vi "G#Interface_ClassToSpecificInterface.vi"(2 "reference in":refnum<class "G#Object.lvclass">, 4 "error in (no error)":errorcluster, 12 "target interface":refnum<class "G#Interface.lvclass">, 14 "autolocate?(F)":bool) -> (22 "interface reference out":refnum<class "G#Interface.lvclass">, 24 "error out":errorcluster)   [LabVIEW 2020, in "G#Interface.lvclass"]
doc: "Casts an ordinary G#Object reference to the specified G#Interface reference."
uses:
  G#Interface.lvclass
  G#Object/G#Object.lvclass
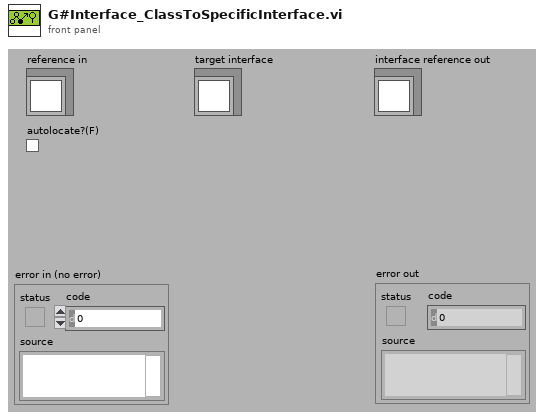
[diagram p1: front panel]
types:
  T1 = typedef "G#Object.lvclass/G#Object_ClassHierarchy.ctl" = cluster{"ClassName":string, "FullClassName":string, "ClassPath":path, "IsLeaf":bool}
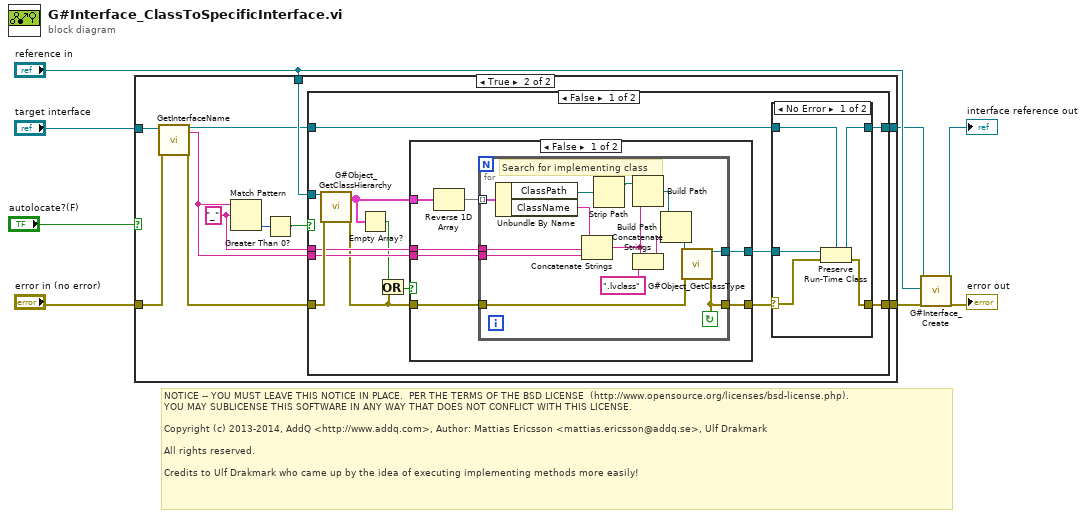
[diagram p0: block diagram]
diagram:
  # "NOTICE -- YOU MUST LEAVE THIS NOTICE IN PLACE.  PER THE TERMS OF THE BSD LICENSE  (http://www.opensource.org/licenses/bsd-license.php).\nYOU MAY SUBLICENSE THIS SOFTWARE IN ANY WAY THAT DOES NOT CONFLICT WITH THIS LICENSE.\n\nCopyright (c) 2013-2014, AddQ <http://www.addq.com>, Author: Mattias Ericsson <mattias.ericsson@addq.se>, Ulf Drakmark\n\nAll rights reserved.\n\nCredits to Ulf Drakmark who came up by the idea of executing implementing methods more easily!"
  n1 = case shown="True" "autolocate?(F)" {
    tunnel: "target interface" -> [w10 w21]
    tunnel: "error in (no error)" -> [w9 w20]
    tunnel: "reference in" -> [_ w19]
    tunnel: [w9 w18] -> w3
    tunnel: [w10 w17] -> w2
    frame False {
    }
    frame True {
      w13 = "_" ("regular expression")
      n2 = call-dynamic "GetInterfaceName.vi"("reference in"=w21, "error in (no error)"=w20) -> ("reference out"=w11:refnum<class "G#Interface.lvclass">, "interface name"=w12:string, "error out"=w15:errorcluster)  [unwired: 13 in, 2 out]
      n3 = Match Pattern(string=w12, regular expression=w13) -> (offset past match=w16:i32)  [unwired: 1 in, 3 out]
      n4 = Greater Than 0?(x=w16) -> (x > 0?=w14:bool)
      n5 = case shown="False" w14 {
        tunnel: w19 -> [w34 _]
        tunnel: w15 -> [w33 w64]
        tunnel: [w29 w64] -> w18
        tunnel: w11 -> [w27 w65]
        tunnel: w13 -> [w32 _]
        tunnel: w12 -> [w31 _]
        tunnel: [w26 w65] -> w17
        frame False {
          n6 = call "G#Object_GetClassHierarchy.vi"("reference in"=w34, "error in (no error)"=w33) -> ("class hierarchy"=w25:T1[], "error out"=w23:errorcluster)  [unwired: 15 in, 1 out]
          n7 = Empty Array?(array=w25) -> (empty?=w24:bool)
          n8 = Or(x=w24, y=w23) -> (x .or. y?=w22:bool)
          n9 = case shown="False" w22 {
            tunnel: w25 -> [w41 _]
            tunnel: w23 -> [w39 w56]
            tunnel: w32 -> [w38 _]
            tunnel: w31 -> [w37 _]
            tunnel: [w36 w56] -> w30
            tunnel: [w35 _] -> w28
            frame False {
              n10 = Reverse 1D Array(array=w41) -> (reversed array=w40:T1[])
              n11 = for {
                tunnel: w40 -> [w55] mode=indexing
                tunnel: w39 -> [w44]
                tunnel: w38 -> [w51]
                tunnel: w37 -> [w50]
                tunnel: [w43] -> w36
                tunnel: [w42] -> w35
                stop <- w43 continue-if-true
                # "Search for implementing class"
                n12 = Unbundle By Name(w55) -> ("ClassPath"=w54:path, "ClassName"=w52:string)
                n13 = Concatenate Strings(w52, w51, w50) -> (w49:string)
                n14 = Strip Path(path=w54) -> (stripped path=w53:path)  [unwired: 1 out]
                n15 = Build Path(base path=w53, name or relative path=w49) -> (appended path=w47:path)
                n16 = Concatenate Strings(w49, ".lvclass" ("string")) -> (w46:string)
                n17 = Build Path(base path=w47, name or relative path=w46) -> (appended path=w45:path)
                n18 = call "G#Object_GetClassType.vi"("class path"=w45, "error in (no error)"=w44) -> ("reference out"=w42:refnum<class "G#Object.lvclass">, "error out"=w43:errorcluster)  [unwired: 16 in]
              }
            }
            frame True {
            }
          }
          n19 = case shown="No Error" w30 {
            selector: w30 -> [w61 w62]
            tunnel: [w60 w62] -> w29
            tunnel: w28 -> [w59 _]
            tunnel: w27 -> [w58 w63]
            tunnel: [w57 w63] -> w26
            frame No Error {
              n20 = Preserve Run-Time Class(object in=w59, error in=w61, 2:w58) -> (object out=w57:refnum<class "G#Interface.lvclass">, error out=w60:errorcluster)
            }
            frame Error {
            }
          }
        }
        frame True {
          # "Implementation interface has been set directly"
        }
      }
    }
  }
  n21 = call-dynamic "G#Interface_Create.vi"("reference in"=w2, "G#Object in"="reference in", "error in (no error)"=w3) -> ("reference out"=→"interface reference out":refnum<class "G#Interface.lvclass">, "error out"=→"error out":errorcluster)  [unwired: 15 in]
